vi "Fib formula node time.vi"() -> ()   [LabVIEW 2013]
panel:
  out "Time ms":u32
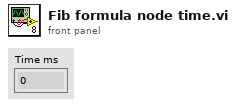
[diagram p1: front panel]
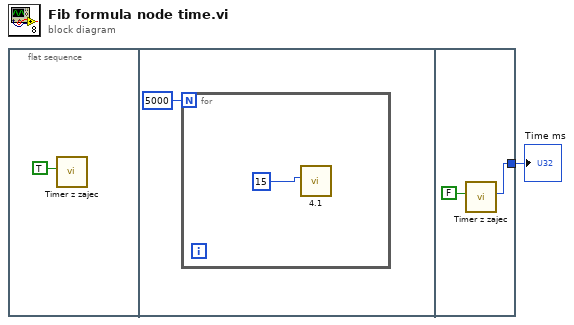
[diagram p0: block diagram]
diagram:
  n1 = flat-sequence {
    tunnel: [w5] -> w1
    frame #0 {
      n2 = call "Timer z zajec.vi"("T start/ F stop"=TRUE) -> ()  [unwired: 10 in, 1 out]
    }
    frame #1 {
      n3 = for {
        N: 5000 -> [_]
        n4 = call "4.1.vi"("input variable"=u32 15 ("n")) -> ()  [unwired: 10 in, 1 out]
      }
    }
    frame #2 {
      n5 = call "Timer z zajec.vi"("T start/ F stop"=FALSE) -> ("Time ms"=w5:u32)  [unwired: 10 in]
    }
  }
  "Time ms" <- w1
